vi "forceConsumerLoop.vi"(8 "error in (no error)":errorcluster) -> (0 "error out":errorcluster)   [LabVIEW 2017, in "externalAquisition.lvlib"]
doc: "This VI is theforce consumer, which connverts the Hall Effects Sensor readings to Fx and Fy using a Neural Network.\n\nThe forcess are written to the 'All data' FGV."
uses:
  externalAquisition.lvlib
  internalQueue/TypeDefs/QueueCommands.ctl
  ErrorMonitor/ErrorMonitor.lvlib
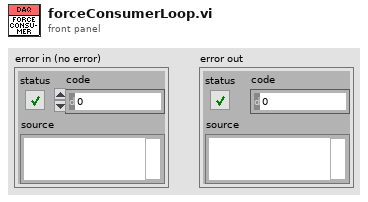
[diagram p1: front panel]
types:
  T1 = typedef "externalAquisition.lvlib/QueueCommands.ctl" = enum16{"obtain", "enqueue", "dequeue", "release"}
  T2 = typedef "dataOut.ctl" = cluster{"X0pos":dbl, "Y0pos":dbl, "Z0pos":dbl, "Fx":dbl, "Fy":dbl, "Fz":dbl, "Encoder1":i32, "Encoder2":i32, "Pot1":dbl, "Pot2":dbl, "Theta0":dbl, "Theta1":dbl, "X1pos":dbl, "Y1pos":dbl, "Z1pos":dbl, "X2pos":dbl, "Y2pos":dbl, "Z2pos":dbl, "ErrorOccurred":bool}
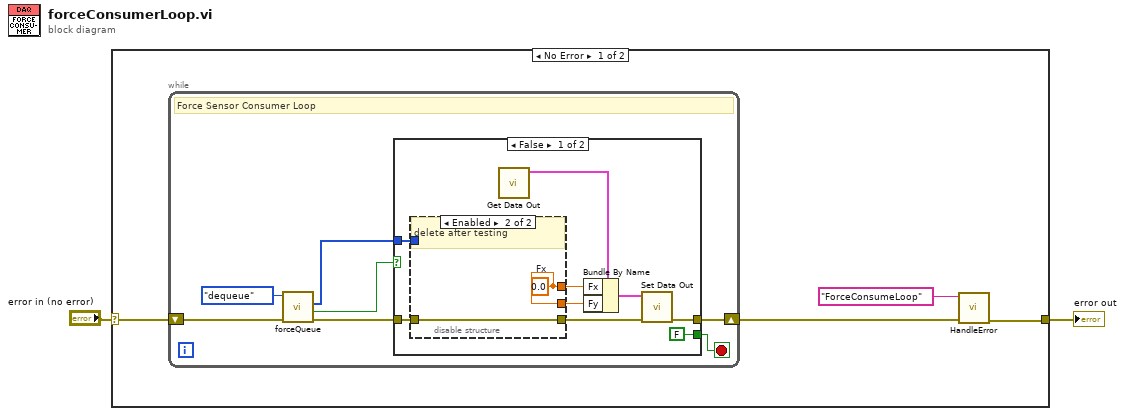
[diagram p0: block diagram]
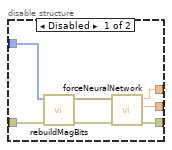
[diagram p2: hidden frame]
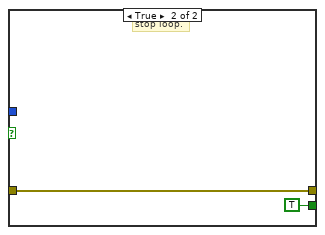
[diagram p3: hidden frame]
diagram:
  n1 = case shown="No Error" "error in (no error)" {
    selector: "error in (no error)" -> [w6 w34]
    tunnel: [w4 w34] -> w2
    frame No Error {
      n2 = while {
        shift-right: [w11] -> w5
        shift-left: w6 -> [w12]
        stop <- w9 stop-if-true
        # "Force Sensor Consumer Loop"
        n3 = call "forceQueue.vi"("error in (no error)"=w12, "Command"=QueueCommands."dequeue") -> ("error out"=w10:errorcluster, "Stop"=w8:bool, "ByteArrayOut"=w7:u8[])  [unwired: 7 in]
        n4 = case shown="False" w8 {
          tunnel: w10 -> [w20 w33]
          tunnel: [w21 w33] -> w11
          tunnel: [FALSE TRUE] -> w9
          tunnel: w7 -> [w19 _]
          frame False {
            n5 = disable-structure shown="Enabled" {
              disable-tunnel: w20 -> [w29 w31]
              disable-tunnel: w19 -> [w28 _]
              disable-tunnel: [w26 w31] -> w18
              disable-tunnel: [w24 w30] -> w15
              disable-tunnel: [w23 w30] -> w14
              frame Disabled {
                n6 = call "rebuildMagBits.vi"("error in (no error)"=w29, "ByteArrayIn"=w28) -> ("error out"=w27:errorcluster, "rawBits"=w25:cluster{u16, u16, u16, u16})  [unwired: 8 in]
                n7 = call "forceNeuralNetwork.vi"("error in (no error)"=w27, "rawBits"=w25) -> ("error out"=w26:errorcluster, "Fy"=w23:dbl, "Fx"=w24:dbl)  [unwired: 7 in]
              }
              frame Enabled {
                w30 = 0.0  # Fx
                # "delete after testing"
              }
            }
            n8 = call "Get Data Out.vi"() -> ("DataOut"=w17:T2)  [unwired: 10 in, 1 out]
            n9 = Bundle By Name(cluster=w17, "Fx"=w15, "Fy"=w14) -> (w16:T2)
            n10 = call "Set Data Out.vi"("error in (no error)"=w18, "DataOut"=w16) -> ("error out"=w21:errorcluster)  [unwired: 9 in]
          }
          frame True {
            # "stop loop."
          }
        }
      }
      n11 = call "HandleError.vi"("error in (no error)"=w5, "Source"="ForceConsumeLoop") -> ("error out"=w4:errorcluster)  [unwired: 9 in]
    }
    frame Error {
    }
  }
  "error out" <- w2
